vi "setFrequency.vi"(8 "error in (no error)":errorcluster, 9 "Frequency (Hz)":dbl, 10 "Channel":i32=1 min=1 max=16, 11 "Instrument.SignalGenerator in":refnum<class "Instrument.SignalGenerator.lvclass">) -> (0 "error out":errorcluster, 3 "Instrument.SignalGenerator out":refnum<class "Instrument.SignalGenerator.lvclass">)   [LabVIEW 2019, in "Instrument.SignalGenerator.lvclass"]
uses:
  Instrument.SignalGenerator.lvclass
  C:/Users/patrick/Documents/GitHub/Instrument-Framework/lvsrc/Framework/Instrument/Instrument.lvclass
  Typedefs/SignalGenerator.Commands--Enum.ctl
  Typedefs/setFloatParameter--enum.ctl
  Instrument/Instrument.lvclass
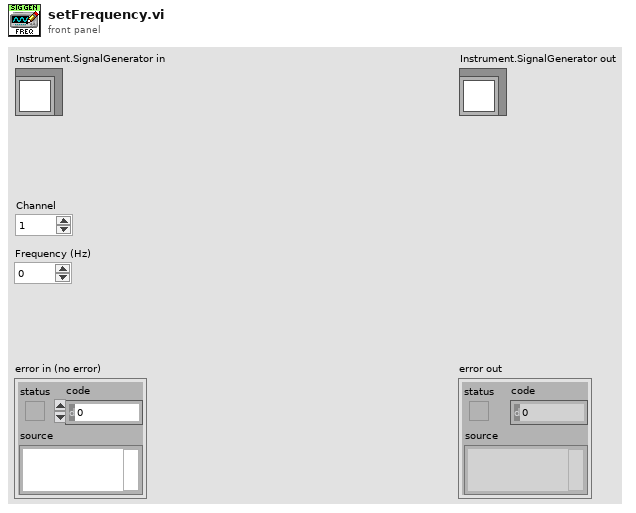
[diagram p1: front panel]
types:
  T1 = typedef "Instrument.SignalGenerator.lvclass/setFloatParameter--enum.ctl" = cluster{"Channel":i32, "Parameter":dbl}
  T2 = typedef "Instrument.SignalGenerator.lvclass/SignalGenerator.Commands--Enum.ctl" = enum16{"setFrequency", "setFunction", "setLevel", "setOffset", "setPhase", "setPower"}
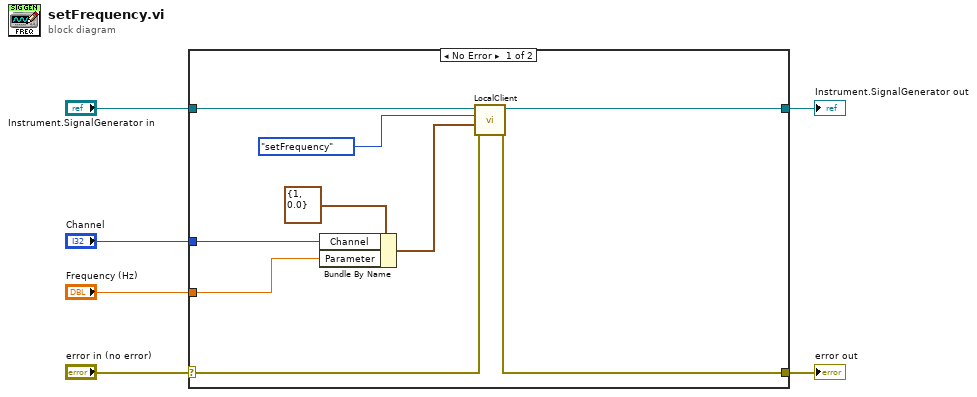
[diagram p0: block diagram]
diagram:
  n1 = case shown="No Error" "error in (no error)" {
    selector: "error in (no error)" -> [w7 w17]
    tunnel: [w13 w17] -> w6
    tunnel: [w14 w16] -> w4
    tunnel: "Instrument.SignalGenerator in" -> [w15 w16]
    tunnel: "Frequency (Hz)" -> [w11 _]
    tunnel: "Channel" -> [w10 _]
    frame No Error {
      n2 = Bundle By Name(cluster=T1 {"Channel"=1, "Parameter"=0.0} ("setFloatParameter"), "Channel"=w10, "Parameter"=w11) -> (w9:T1)
      n3 = call "LocalClient.vi"("timeout (ms) [500]"=SignalGenerator.Commands--Enum."setFrequency" ("Commands"), "error in (no error)"=w7, "params"=w9, "Instrument in"=w15) -> ("error out"=w13:errorcluster, "Instrument out"=w14:refnum<class "Instrument.SignalGenerator.lvclass">)  [unwired: 4 in, 2 out]
    }
    frame Error {
    }
  }
  "error out" <- w6
  "Instrument.SignalGenerator out" <- w4
